vi "local.Initialize (NVMEM Area).vi"(0 "NVMEM areas":refnum<k21>, 7 "reservation access (Read/Write)":i32(ring)=3 items=["None"=0, "Read Only"=1, "Read/Write"=3], 9 "reservation group":string, 11 "error in (no error)":errorcluster, 12 "connect timeout (60 sec)":dbl=60.0) -> (4 "SLSC Local out":refnum<class "SLSC Local.lvclass">, 15 "error out":errorcluster)   [LabVIEW 2016, in "SLSC Interfaces.lvlib" / "SLSC Local.lvclass"]
uses:
  SLSC Local.lvclass
  <vilib>/SLSC/SLSC.lvlib
  <vilib>/SLSC/Initialize Session with NVMEM Areas.vi
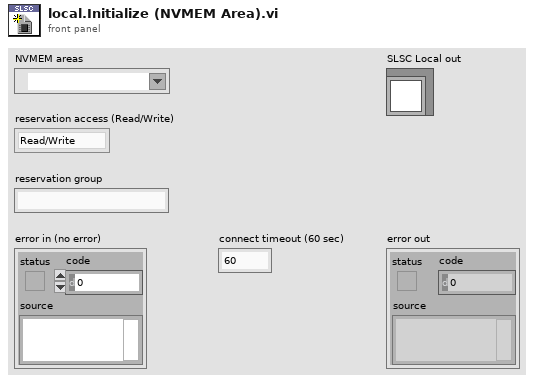
[diagram p1: front panel]
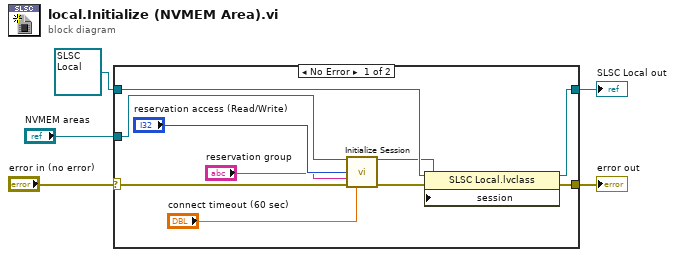
[diagram p0: block diagram]
diagram:
  n1 = case shown="No Error" "error in (no error)" {
    selector: "error in (no error)" -> [w15 w17]
    tunnel: [w6 w17] -> w4
    tunnel: [w7 w16] -> w2
    tunnel: refnum<class "SLSC Local.lvclass"> refnum ("SLSC Local in") -> [w10 w16]
    tunnel: "NVMEM areas" -> [w11 _]
    frame No Error {
      n2 = call-poly <vilib>:"Initialize Session.vi"("NVMEM areas"=w11, "reservation access (Read/Write)"="reservation access (Read/Write)", "reservation group"="reservation group", "error in (no error)"=w15, "connect timeout (60 sec)"="connect timeout (60 sec)") -> ("session out"=w8:refnum<k21>, "error out"=w9:errorcluster)  [unwired: 9 in]
      n3 = property class="SLSC Local.lvclass"(reference=w10, error in=w9, "session"=w8) -> (reference out=w7:refnum<class "SLSC Local.lvclass">, error out=w6:errorcluster)
    }
    frame Error {
    }
  }
  "error out" <- w4
  "SLSC Local out" <- w2
